vi "read_H2_N2.vi"() -> (0 "H2N2 Flow Rate":dbl, 1 "Remote":bool, 2 "Display H2N2":bool, 3 "N2 Active":bool, 4 "H2 Active":bool)   [LabVIEW 2011]
uses:
  low_level_proc/globals.vi
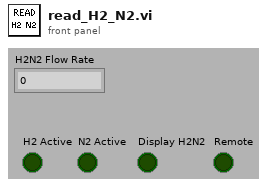
[diagram p1: front panel]
types:
  T1 = typedef "relaySpec.ctl" = cluster{"Card Index":u16, "Relay Index":u16}
  T2 = typedef "DA_Spec.ctl" = cluster{"Card Index":u16, "Channel Index":u16}
  T3 = typedef "AD_Spec.ctl" = u16
  T4 = cluster{"Relay Functions":cluster{"Remote":T1, "H2 active":T1, "N2 active":T1, "Output":T1}, "D/A Functions":cluster{"H2 flow":T2, "N2 flow":T2}, "Flow Ranges":cluster{"H2 flow (HMFC1)":u16, "N2 flow (NMFC1)":u16}, "A/D Functions":cluster{"H2/N2 flow":T3}}
  T5 = cluster{"Remote":T1, "H2 active":T1, "N2 active":T1, "Output":T1}
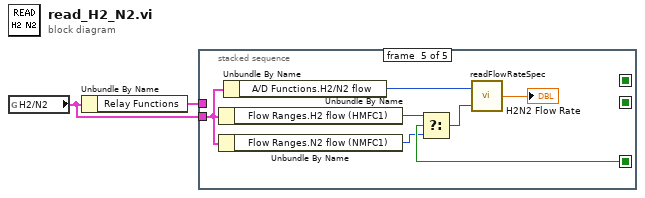
[diagram p0: block diagram]
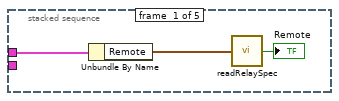
[diagram p2: hidden frame]
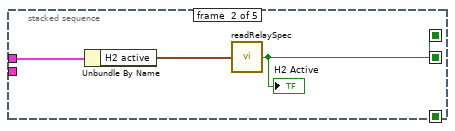
[diagram p3: hidden frame]
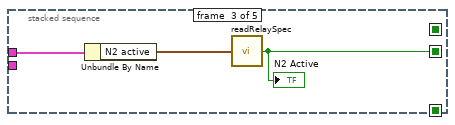
[diagram p4: hidden frame]
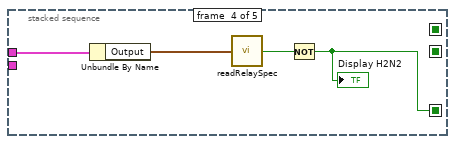
[diagram p5: hidden frame]
diagram:
  n1 = global read "globals.vi" "H2/N2"() -> (w1:T4)
  n2 = Unbundle By Name(w1) -> ("Relay Functions"=w2:T5)
  n3 = stacked-sequence {
    seq-local: [_ w6 _ _ _] -> [_ _ _ _ _]
    seq-local: [_ _ w9 _ _] -> [_ _ _ _ _]
    seq-local: [_ _ _ w15 _] -> [_ _ _ _ w20]
    tunnel: w2 -> [w4 w8 w10 w13 _]
    tunnel: w1 -> [_ _ _ _ w21]
    frame #0 {
      n4 = Unbundle By Name(w4) -> ("Remote"=w3:T1)
      n5 = call "readRelaySpec.vi"("RelaySpec"=w3) -> ("Relay Status"=→"Remote":bool)
    }
    frame #1 {
      n6 = Unbundle By Name(w8) -> ("H2 active"=w7:T1)
      n7 = call "readRelaySpec.vi"("RelaySpec"=w7) -> ("Relay Status"=w6:bool)
      "H2 Active" <- w6
    }
    frame #2 {
      n8 = Unbundle By Name(w10) -> ("N2 active"=w11:T1)
      n9 = call "readRelaySpec.vi"("RelaySpec"=w11) -> ("Relay Status"=w9:bool)
      "N2 Active" <- w9
    }
    frame #3 {
      n10 = Unbundle By Name(w13) -> ("Output"=w14:T1)
      n11 = call "readRelaySpec.vi"("RelaySpec"=w14) -> ("Relay Status"=w12:bool)
      n12 = Not(x=w12) -> (.not. x?=w15:bool)
      "Display H2N2" <- w15
    }
    frame #4 {
      n13 = Unbundle By Name(w21) -> ("Flow Ranges.H2 flow (HMFC1)"=w22:u16)
      n14 = Unbundle By Name(w21) -> ("Flow Ranges.N2 flow (NMFC1)"=w19:u16)
      n15 = Unbundle By Name(w21) -> ("A/D Functions.H2/N2 flow"=w18:T3)
      n16 = Select(t=w22, s=w20, f=w19) -> (s? t:f=w17:u16)
      n17 = call "readFlowRateSpec.vi"("Flow range Index"=w17, "Channel Index"=w18) -> ("Flow Rate (sccm)"=→"H2N2 Flow Rate":dbl)
    }
  }
